vi "Visor_ondas.vi"() -> ()   [LabVIEW 2026]
uses:
  <vilib>/Utility/file.llb/Read Delimited Spreadsheet (string).vi
panel:
  out "XY Graph":cluster{i32[], i32[]}(graph)
  out "subarray 2":i32[](array[numeric])
  out "subarray":i32[](array[numeric])
  out "number":i32[][](array[numeric])
  in  "Leer CSV":bool
  in  "stop":bool
  out "all rows":string[][](array[string])
  in  "Archivo CSV":path
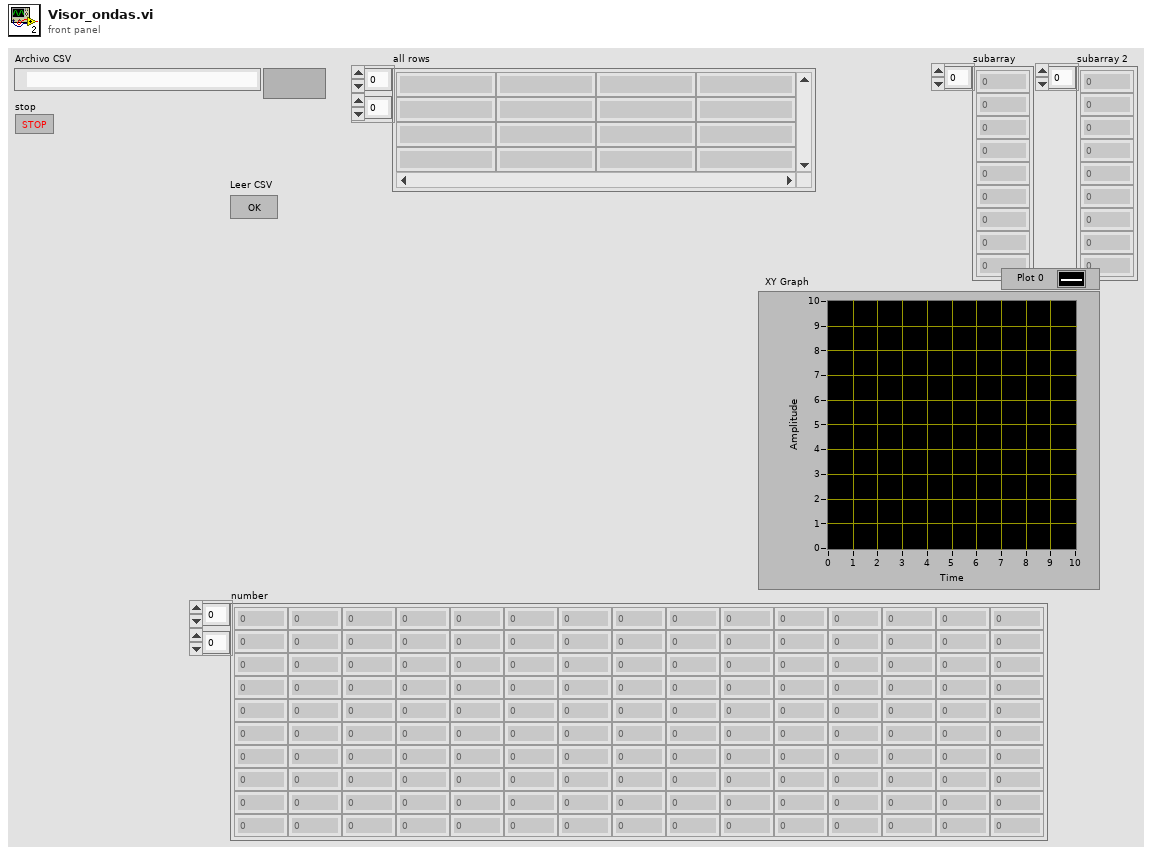
[diagram p1: front panel]
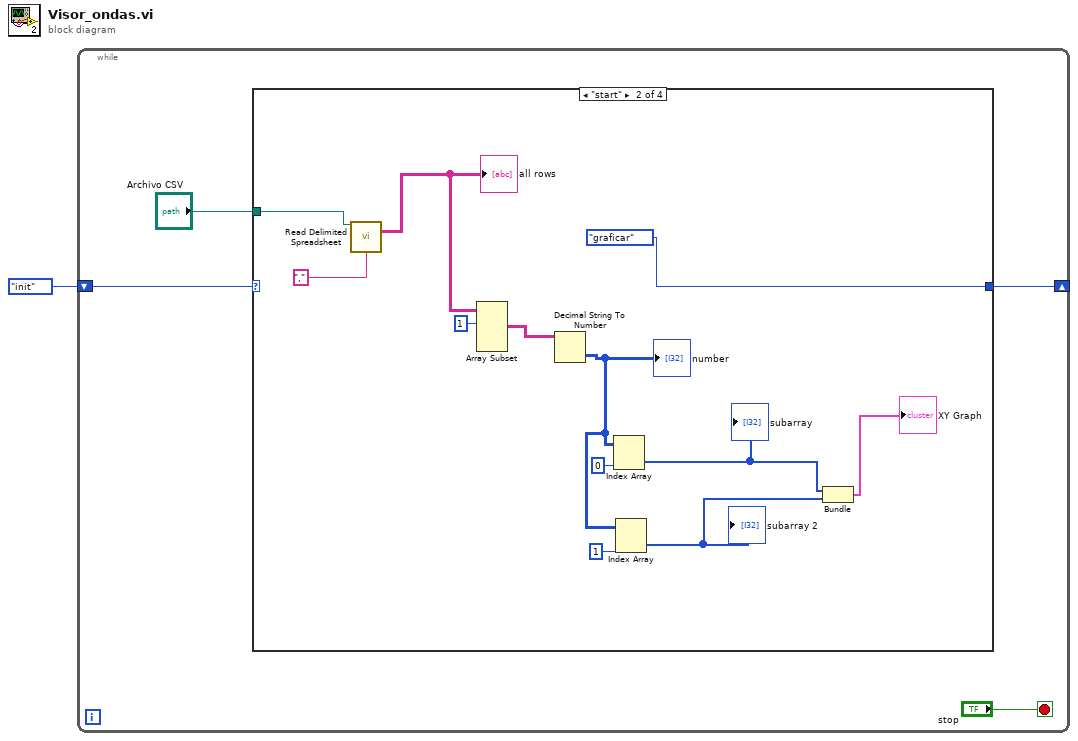
[diagram p0: block diagram]
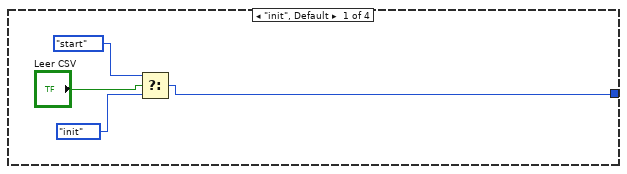
[diagram p2: hidden frame]
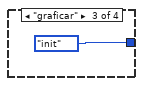
[diagram p3: hidden frame]
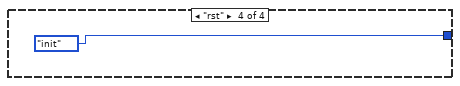
[diagram p4: hidden frame]
diagram:
  n1 = while {
    shift-right: [w2] -> _
    shift-left: enum16{"init", "start", "graficar", "rst"}."init" -> [w3]
    stop <- "stop" stop-if-true
    n2 = case shown="\"start\"" w3 {
      tunnel: "Archivo CSV" -> [_ w20 _ _]
      tunnel: [w6 enum16{"init", "start", "graficar", "rst"}."graficar" enum16{"init", "start", "graficar", "rst"}."init" enum16{"init", "start", "graficar", "rst"}."init"] -> w2
      frame "init", Default {
        n3 = Select(t=enum16{"init", "start", "graficar", "rst"}."start", s="Leer CSV", f=enum16{"init", "start", "graficar", "rst"}."init") -> (s? t:f=w6:enum16{"init", "start", "graficar", "rst"})
      }
      frame "start" {
        n4 = call-poly <vilib>:"Read Delimited Spreadsheet.vi"("file path (dialog if empty)"=w20, "delimiter (\\t)"="," ("delimiter (\\t)")) -> ("all rows"=w18:string[][])  [unwired: 8 in, 5 out]
        "all rows" <- w18
        n5 = Array Subset(array=w18, index (row)=1 ("index")) -> (w16:string[][])  [unwired: 3 in]
        n6 = Decimal String To Number(string=w16) -> (number=w14:i32[][])  [unwired: 2 in, 1 out]
        "number" <- w14
        n7 = Index Array(array=w14, index (col)=0 ("disabled index (col)")) -> (element=w12:i32[])  [unwired: 1 in]
        "subarray" <- w12
        n8 = Index Array(array=w14, index (col)=1 ("disabled index (col)")) -> (element=w11:i32[])  [unwired: 1 in]
        "subarray 2" <- w11
        n9 = Bundle(w12, w11) -> (→"XY Graph":cluster{i32[], i32[]})  [unwired: 1 in]
      }
      frame "graficar" {
      }
      frame "rst" {
      }
    }
  }
